vi "SetEnumSerialPortList.vi"(8 "error in (no error)":errorcluster caption="错误输入（无错误）", 9 "Array":T1(array[cluster])) -> (0 "error out":errorcluster caption="错误输出", 2 "function return":i32)   [LabVIEW 2013, in "MvCameraControl.lvlib"]
doc: "MV_LV_API int __stdcall GetStringValue( void* handle, const char* strKey, MVCC_STRINGVALUE *pStringValue);"
uses:
  MvCameraControl.lvlib
  MvCameraPatch.dll
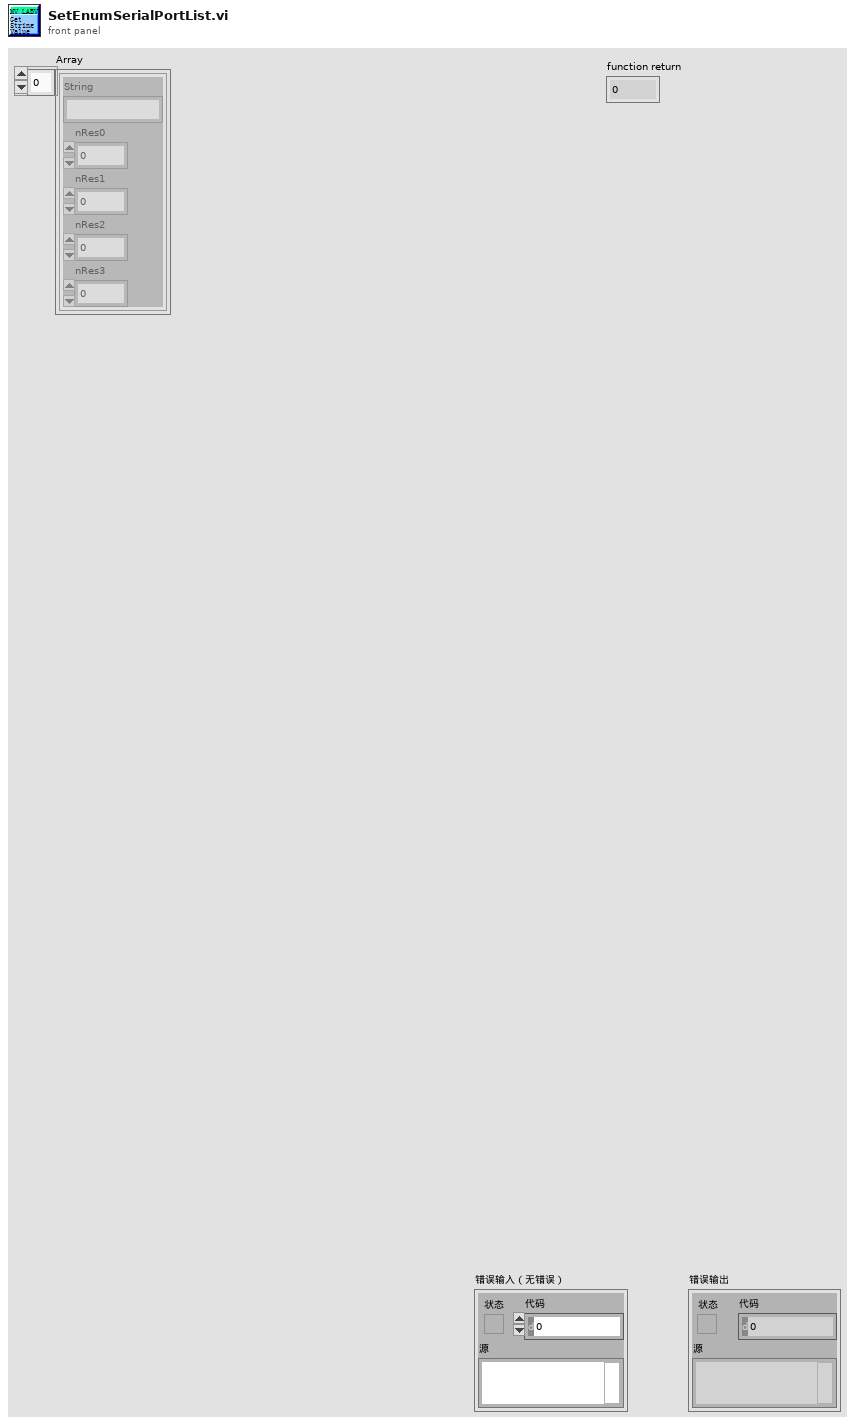
[diagram p1: front panel]
types:
  T1 = cluster{"String":string, "nRes0":u32, "nRes1":u32, "nRes2":u32, "nRes3":u32}[]
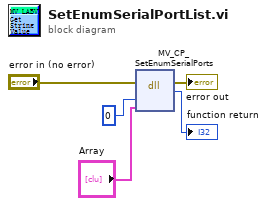
[diagram p0: block diagram]
diagram:
  n1 = dll-call lib="MvCameraPatch.dll" fn="MV_CP_SetEnumSerialPorts"(error in="error in (no error)", "nSerialPortNum"=u32 0, "pSerialPortList"="Array") -> (error out=→"error out":errorcluster, "返回类型"=→"function return":i32)  [unwired: 4 in, 1 out]
